vi "Main.vi"() -> ()   [LabVIEW 2013]
uses:
  Global.vi
  <userlib>/QLC/QLC.lvlib
panel:
  out "Error TCP_quad":errorcluster
  out "TCP_quad ID":refnum<k5>
  in  "Quadcopter":bool
  out "Trailers":bool[](array[boolean])
  out "Platooning Distance Scenario":dbl
  out "Distance2Master Scenario":dbl[](array[numeric])
  out "CurrentWP Final DarkGrey":i32
  out "Vref DarkGrey Final":dbl
  out "CurrentWP Final Grey":i32
  out "Vref Grey Final":dbl
  out "CurrentWP Final Black":i32
  out "Vref Black Final":dbl
  out "CurrentWP Final Blue":i32
  out "Vref Blue Final":dbl
  out "CurrentWP Final Red":i32
  out "Vref Red Final":dbl
  in  "Platooning Speed  Increment":dbl=1.25
  out "StopArrayOuter":i32[](array[numeric])
  out "StopArrayInner":i32[](array[numeric])
  out "PlatoonArray":i32[](array[numeric])
  out "Grey Truck Pose":sgl[](array[numeric])
  out "DarkGrey Truck Pose":dbl[](array[numeric])
  out "Current DarkGrey State":i32
  out "DarkGrey Trajectory WP Out":dbl[][](array[numeric])
  out "Red distance2Master DarkGrey":dbl
  out "DarkGrey dref":dbl
  out "Red distance2Master Grey":dbl
  out "Current Grey State":i32
  out "Grey Trajectory WP Out":dbl[][](array[numeric])
  out "Grey dref":dbl
  out "Change to state DarkGrey Scenario":i32
  out "Vref DarkGrey Scenario":dbl
  out "Change to state Grey Scenario":i32
  out "Vref Grey Scenario":dbl
  in  "ID DarkGrey":u8=5
  in  "ID Grey":u8=4
  in  "Change to state DarkGrey":i32(ring)=1 items=["Parking", "OuterLane", "InnerLane", "InnerRoad"]
  in  "Vref DarkGrey":dbl(slide) scale=0.0..1.5
  in  "Change to state Grey":i32(ring)=1 items=["Parking", "OuterLane", "InnerLane", "InnerRoad"]
  in  "Vref Grey":dbl(slide) scale=0.0..1.5
  out "X Grey":dbl
  out "Y  Grey":dbl
  out "Yaw  Grey":dbl
  out "X DarkGrey":dbl
  out "Y  DarkGrey":dbl
  out "Yaw  DarkGrey":dbl
  in  "ControllerGains DarkGrey":T1={"KPSteering"=1.0, "KDSteering"=0.0, "KPSpeed"=0.8, "KISpeed"=3.0, "KDSpeed"=0.2}
  out "Current state DarkGrey":i32(ring)=1 items=["Parking", "OuterLane", "InnerLane", "InnerRoad"]
  out "D2TL DarkGrey":dbl
  out "D2Master DarkGrey":dbl
  in  "With Trailer DarkGrey":bool
  out "Real Speed DarkGrey":dbl(knob) scale=0.0..2.0
  out "DarkGrey Speed":u8
  out "DarkGrey Steering":u8
  in  "ControllerGains Grey":T1={"KPSteering"=0.6, "KDSteering"=0.05, "KPSpeed"=0.8, "KISpeed"=3.0, "KDSpeed"=0.2}
  out "Current state Grey":i32(ring)=1 items=["Parking", "OuterLane", "InnerLane", "InnerRoad"]
  out "D2TL Grey":dbl
  out "D2Master Grey":dbl
  in  "With Trailer Grey":bool
  out "Real Speed Grey":dbl(knob) scale=0.0..2.0
  out "Grey Speed":u8
  out "Grey Steering":u8
  out "COM  DarkGrey":T2
  out "COM  Grey":T2
  in  "DarkGrey ID":u8=9
  in  "Grey ID":u8=8
  in  "Port DarkGrey":u16=9006
  in  "Port Grey":u16=9005
  in  "QTM ID DarkGrey":i32=3
  in  "QTM ID Grey":i32=5
  out "Vref":dbl[](array[numeric])
  out "bytes written 3":i32
  out "bytes written 2":i32
  out "ScenarioString":string
  out "red dref":dbl
  out "real distance2master red":dbl
  in  "ControllerGains Black":T1={"KPSteering"=0.9, "KDSteering"=0.05, "KPSpeed"=1.0, "KISpeed"=3.0, "KDSpeed"=0.2}
  in  "ControllerGains Blue":T1={"KPSteering"=1.0, "KDSteering"=0.05, "KPSpeed"=0.8, "KISpeed"=3.0, "KDSpeed"=0.2}
  out "Version":i32
  in  "Visualizer":bool
  out "Iter":i32
  out "NRoads":i32
  out "TL Outer Select":bool
  out "TL Inner Select":bool
  out "Error TCP":errorcluster
  out "TCP ID":refnum<k5>
  out "NTrucks":i32
  out "CurrentWP":i32[](array[numeric])
  out "Last QTM Event":dbl=2.0
  out "Change to state Red Scenario":i32
  out "Vref Red Scenario":dbl
  out "Change to state Blue Scenario":i32
  out "Vref Blue Scenario":dbl
  out "Change to state Black Scenario":i32
  out "Vref Black Scenario":dbl
  out "Ignore":bool
  out "Current state Red":i32(ring)=1 items=["Parking", "OuterLane", "InnerLane", "InnerRoad"]
  out "Current state Blue":i32(ring)=1 items=["Parking", "OuterLane", "InnerLane", "InnerRoad"]
  out "Current state Black":i32(ring)=1 items=["Parking", "OuterLane", "InnerLane", "InnerRoad"]
  in  "Tab Control":enum32{"Pedro Lima", "João Pedro Alvito"}(tab)
  in  "Scenario Selection PL":u32(ring) items=["Manual", "1 catch up 1", "1 catch up 2", "2 catch up 1", "1 catch up 1 from other road", "1 catch up 1 but master exits", "1 diferent mass catch up 2 without overtake", "1 different mass catch up 2 with overtake", "1 catch up 2 but middle leaves"]
  out "Info PL":string
  out "length":i32
  in  "Bridge":bool
  in  "Scenario Selection JPA":u32(ring) items=["Manual", "Simple traffic lights", "Simple anti-platoon", "Mixture", "Time Decision", "Timed Control with Platoon", "Anti-platoon"]
  out "Info JP":string
  out "X Red":dbl
  out "Y  Red":dbl
  out "Yaw  Red":dbl
  out "X Black":dbl
  out "Y Black":dbl
  out "Yaw Black":dbl
  out "Yaw Blue":dbl
  out "Y Blue":dbl
  out "X Blue":dbl
  out "D2TL Red":dbl
  out "D2TL Black":dbl
  out "D2TL Blue":dbl
  out "D2Master Red":dbl
  out "D2Master Black":dbl
  out "D2Master Blue":dbl
  out "Outer Red":bool
  out "Inner Green":bool
  out "Inner Red":bool
  out "Outer Green":bool
  out "D2TLFinal":dbl[](array[numeric])
  out "Truck Dimensions":dbl[](array[numeric])
  out "Traffic Lights":T3
  in  "Stop Button Inner":bool
  in  "Traffic Light Position Inner Lane":i32=23
  out "CurrentState":i32[](array[numeric])
  out "Real Speed Red":dbl(knob) scale=0.0..2.0
  out "Real Speed Black":dbl(knob) scale=0.0..2.0
  in  "Stop Button Outer":bool
  in  "Traffic Light Position Outer Lane":i32=27
  out "InnerRoad":T4
  out "Distance to Master":dbl[](array[numeric])
  out "Blue dref":dbl
  out "Blue distance2master blue":dbl
  out "black dref":dbl
  out "Red distance2Master black":dbl
  out "Red Trajectory WP Out":dbl[][](array[numeric])
  out "Blue Trajectory WP Out":dbl[][](array[numeric])
  out "Black Trajectory WP Out":dbl[][](array[numeric])
  in  "Change to state Black":i32(ring)=1 items=["Parking", "OuterLane", "InnerLane", "InnerRoad"]
  in  "Change to state Red":i32(ring)=1 items=["Parking", "OuterLane", "InnerLane", "InnerRoad"]
  out "Trajectory Network":T5(array[cluster])
  out "InnerLane":T4
  out "OuterLane":T4
  out "Current Red State":i32
  out "Current Black State":i32
  out "Current Blue State":i32
  in  "Change to state Blue":i32(ring)=1 items=["Parking", "OuterLane", "InnerLane", "InnerRoad"]
  out "Trucks Poses":dbl[][](array[numeric])
  out "Total Platooning Distance":dbl[](array[numeric])
  in  "With Trailer Red":bool
  in  "With Trailer  Black":bool
  in  "With Trailer Blue":bool
  in  "QTM ID Red":i32=4
  in  "QTM ID Blue":i32=2
  in  "QTM ID Black":i32=1
  in  "ID Black":u8=2
  in  "ID Red":u8=3
  in  "ID Blue":u8=1
  out "COM  Black":T2
  out "COM  Red":T2
  out "COM Blue":T2
  in  "Platooning Distance":dbl=0.3
  out "Distance2Master":dbl[](array[numeric])
  out "Real Speed Blue":dbl(knob) scale=0.0..2.0
  in  "Set MasterID":i32(ring) items=["None", "Blue Truck", "Black Truck", "Red Truck", "Grey Truck", "DarkGrey Truck"]
  in  "Vref Black":dbl(slide) scale=0.0..1.5
  in  "Vref Blue":dbl(slide) scale=0.0..1.5
  in  "Vref Red":dbl(slide) scale=0.0..1.5
  out "Red Truck Pose":dbl[](array[numeric])
  out "Blue Truck Pose":dbl[](array[numeric])
  out "Black Truck Pose":dbl[](array[numeric])
  out "Red Speed":u8
  out "Red Steering":u8
  in  "Event Label":string
  in  "Set Event":bool
  in  "stop":bool
  out "Blue Speed":u8
  out "Blue Steering":u8
  in  "Port Blue":u16=9002
  in  "Blue ID":u8=10
  out "Camera Timestamp":u64
  out "Camera Frame Number":u32
  in  "Control QTM":bool caption="Off   On"
  out "Controlling QTM":bool
  in  "Connect to QTM":bool=TRUE
  out "QTM Message":string
  in  "Data":string="6DEuler"
  in  "Frequency":string="AllFrames"
  in  "Port":i32=22222 min=22222 max=65535
  in  "Address":string="smlremote.no-ip.biz"
  in  "Port Red":u16=9004
  in  "Red ID":u8=7
  out "Black Speed":u8
  out "Black Steering":u8
  in  "Port Black":u16=9003
  in  "Black ID":u8=14
  in  "ControllerGains Red":T1={"KPSteering"=1.0, "KDSteering"=0.05, "KPSpeed"=0.8, "KISpeed"=3.0, "KDSpeed"=0.2}
types:
  T1 = cluster{"KPSteering":dbl, "KDSteering":dbl, "KPSpeed":dbl, "KISpeed":dbl, "KDSpeed":dbl}
  T2 = cluster{"Truck ID":u8, "connection ID":refnum<k5>}
  T3 = cluster{"Stop Button Outer":bool, "Stop WP Outer Lane":dbl, "Stop Button Inner":bool, "Stop WP Inner Lane ":dbl}
  T4 = cluster{"all rows":dbl[][], "all rows":dbl[][], "Array":i32[]}
  T5 = cluster{"Trajectory WP":dbl[][], "Distances LUT":dbl[][], "Trajectory length":i32[]}[]
  T6 = cluster{"pose":dbl[], "totalerror_v":dbl, "erroSteering":dbl, "ActualTime":dbl, "ActualTime 2":dbl}
  T7 = cluster{"all rows":dbl[][], "all rows":dbl[][], "Array":i32[]}[]
  T8 = cluster{"Trajectory WP":dbl[][], "Distances LUT":dbl[][], "Trajectory length":i32[]}
  T9 = cluster{"Vref Black":dbl, "Change to state Black":i32, "Vref Blue":dbl, "Change to state Blue":i32, "Vref Red":dbl, "Change to state Red":i32, "Vref Grey":dbl, "Change to state Grey":i32, "Vref DarkGrey":dbl, "Change to state DarkGrey":i32, "With Trailer Blue":bool, "With Trailer  Black":bool, "With Trailer Red":bool, "With Trailer Grey":bool, "With Trailer DarkGrey":bool, "Platooning Distance":dbl, "CurrentWP":i32[], "Distance to Master":dbl[], "D2TLFinal":dbl[], "CurrentState":i32[], "Trajectory Network":cluster{"Trajectory WP":dbl[][], "Distances LUT":dbl[][], "Trajectory length":i32[]}[]}
  T10 = cluster{"Vref_Black":dbl, "Change_to_state_Black":i32, "Vref_Blue":dbl, "Change_to_state_Blue":i32, "Vref_Red":dbl, "Change_to_state_Red":i32, "Vref_Grey":dbl, "Change_to_state_Grey":i32, "Vref_DarkGrey":dbl, "Change_to_state_DarkGrey":i32, "With_Trailer_Blue":bool, "With_Trailer_Black":bool, "With_Trailer_Red":bool, "With_Trailer_Grey":bool, "With_Trailer_DarkGrey":bool, "Platooning_Distance":dbl, "CurrentWP":i32[], "Distance2Master":dbl[], "d2TL":dbl[], "CurrentState":i32[], "TrajectoryNetwork":cluster{"TrajectoryWP":dbl[][], "DistancesLUT":dbl[][], "TrajectoryLength":i32[]}[]}
  T11 = cluster{"Stop Button Outer":bool, "Traffic Light Position Outer Lane":i32, "Stop Button Inner":bool, "Traffic Light Position Inner Lane":i32}
  T12 = cluster{"pose":dbl[], "totalerror_v":dbl, "erroSteering":dbl, "ActualTime":dbl, "error_v":dbl}
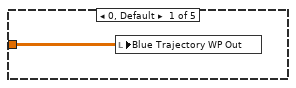
[diagram p5: hidden frame]
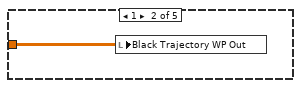
[diagram p6: hidden frame]
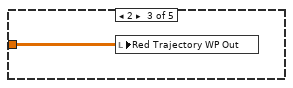
[diagram p7: hidden frame]
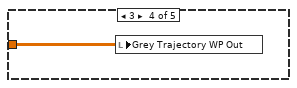
[diagram p8: hidden frame]
diagram:
  n1 = flat-sequence {
    frame #0 {
      n2 = flat-sequence {
        frame #0 {
          n3 = call "CreateConnection.vi"("Truck ID"="DarkGrey ID", "Port number\nactuators"="Port DarkGrey") -> ("COM data"=→"COM  DarkGrey":T2)  [unwired: 1 in]
          n4 = call "CreateConnection.vi"("Truck ID"="Red ID", "Port number\nactuators"="Port Red") -> ("COM data"=→"COM  Red":T2)  [unwired: 1 in]
          n5 = call "CreateConnection.vi"("Truck ID"="Black ID", "Port number\nactuators"="Port Black") -> ("COM data"=→"COM  Black":T2)  [unwired: 1 in]
          n6 = call "CreateConnection.vi"("Truck ID"="Blue ID", "Port number\nactuators"="Port Blue") -> ("COM data"=→"COM Blue":T2)  [unwired: 1 in]
          n7 = call "CreateConnection.vi"("Truck ID"="Grey ID", "Port number\nactuators"="Port Grey") -> ("COM data"=→"COM  Grey":T2)  [unwired: 1 in]
        }
      }
      n8 = flat-sequence {
        frame #0 {
          # "Initializations"
          n9 = Build Array(0 ("element"), 0 ("element"), 0 ("element"), 0 ("element"), 0 ("element")) -> (w78:i32[])
          "CurrentState" <- w78
          n10 = Build Array(0 ("element"), 0 ("element"), 0 ("element"), 0 ("element"), 0 ("element")) -> (→"CurrentWP":i32[])
          n11 = global write "Global.vi" "Transition WP"(i32[][] [[-1, -1, -1, -1], [-1, -1, -1, -1], [-1, -1, 5, 1], [-1, -1, 50, 25]] ("Transition WP")) -> ()
          n12 = global write "Global.vi" "RealSpeed"(dbl[] [] ("RealSpeed")) -> ()
          n13 = Build Array("Tab Control", "Scenario Selection PL", "Scenario Selection JPA") -> (w59:u32[])
          n14 = global write "Global.vi" "ScenarioArray"(w59) -> ()
          n15 = Array Size(array=w78) -> (size(s)=→"NTrucks":i32)
          n16 = local write "Set MasterID"(0 ("MasterID")) -> ()
          n17 = global write "Global.vi" "IsOvertaking"(FALSE ("IsOvertaking")) -> ()
          n18 = Index Array(array=w59, index=0) -> (element=w60:u32)
          n19 = global write "Global.vi" "Positioned"(FALSE ("FirstTime")) -> ()
          n20 = global write "Global.vi" "MasterID"(0 ("MasterID")) -> ()
          n21 = Increment(x=w60) -> (x+1=w61:u32)
          n22 = global write "Global.vi" "stop"(FALSE ("stop")) -> ()
          n23 = Index Array(array=w59, index=w61) -> (element=w62:u32)
          n24 = global write "Global.vi" "TL  Inner"(FALSE ("TL  Inner")) -> ()
          n25 = global write "Global.vi" "TL Outer"(FALSE ("TL Outer")) -> ()
          n26 = global write "Global.vi" "Lap Counter"(0 ("Lap Counter")) -> ()
          n27 = global write "Global.vi" "FirstTime"(TRUE ("FirstTime")) -> ()
          n28 = Not Equal To 0?(x=w62) -> (x != 0?=→"Ignore":bool)
          n29 = global write "Global.vi" "SetMasterID"(0 ("MasterID")) -> ()
          "ScenarioString" <- " " ("ScenarioString")
          "Vref" <- dbl[] [] ("RealSpeed")
        }
      }
      n30 = flat-sequence {
        frame #0 {
          n31 = local read "Tab Control"() -> (w2:enum32{"Pedro Lima", "João Pedro Alvito"})
          n32 = call "GetVersion.vi"() -> ("number"=→"Version":i32)
          n33 = Not Equal To 0?(x=w2) -> (x != 0?=w1:bool)
          n34 = local read "Version"() -> (w7:i32)
          n35 = local read "Version"() -> (w8:i32)
          n36 = local read "Version"() -> (w9:i32)
          n37 = local read "Version"() -> (w10:i32)
          n38 = local read "Version"() -> (w12:i32)
          n39 = local read "Version"() -> (w14:i32)
          n40 = local read "Version"() -> (w6:i32)
          n41 = local read "Version"() -> (w13:i32)
          n42 = call "CreatePath.vi"("Matlab Version"=w7, "filename"="OuterLaneBridgeLUT.txt") -> ("FinalPath"=w20:path)
          n43 = call "CreatePath.vi"("Matlab Version"=w8, "filename"="OuterLaneLUT.txt") -> ("FinalPath"=w22:path)
          n44 = call "CreatePath.vi"("Matlab Version"=w9, "filename"="OuterLaneBridge.txt") -> ("FinalPath"=w24:path)
          n45 = call "CreatePath.vi"("Matlab Version"=w10, "filename"="OuterLane.txt") -> ("FinalPath"=w26:path)
          n46 = call "CreatePath.vi"("Matlab Version"=w12, "filename"="InnerLaneBridgeLUT.txt") -> ("FinalPath"=w34:path)
          n47 = call "CreatePath.vi"("Matlab Version"=w14, "filename"="InnerLaneLUT.txt") -> ("FinalPath"=w33:path)
          n48 = call "CreatePath.vi"("Matlab Version"=w6, "filename"="InnerLaneBridge.txt") -> ("FinalPath"=w30:path)
          n49 = call "CreatePath.vi"("Matlab Version"=w13, "filename"="InnerLane.txt") -> ("FinalPath"=w28:path)
          n50 = local read "Version"() -> (w11:i32)
          n51 = local read "Version"() -> (w15:i32)
          n52 = And(x="Bridge", y=w1) -> (x .and. y?=w4:bool)
          n53 = call "CreatePath.vi"("Matlab Version"=w11, "filename"="InnerRoadLUT.txt") -> ("FinalPath"=w16:path)
          n54 = call "CreatePath.vi"("Matlab Version"=w15, "filename"="InnerRoad.txt") -> ("FinalPath"=w18:path)
          n55 = Select(t=w20, s=w4, f=w22) -> (s? t:f=w41:path)
          n56 = Select(t=w24, s=w4, f=w26) -> (s? t:f=w40:path)
          n57 = Select(t=w34, s=w4, f=w33) -> (s? t:f=w38:path)
          n58 = Select(t=w30, s=w4, f=w28) -> (s? t:f=w39:path)
          n59 = call "ReadFromFile.vi"("Trajectory Path File"=w40, "Trajectory Distances LUT"=w41) -> ("Trajectory Data"=w45:T4)  [unwired: 1 in]
          "OuterLane" <- w45
          n60 = call "ReadFromFile.vi"("Trajectory Path File"=w18, "Trajectory Distances LUT"=w16) -> ("Trajectory Data"=w42:T4)  [unwired: 1 in]
          "InnerRoad" <- w42
          n61 = call "ReadFromFile.vi"("Trajectory Path File"=w39, "Trajectory Distances LUT"=w38) -> ("Trajectory Data"=w44:T4)  [unwired: 1 in]
          "InnerLane" <- w44
          n62 = Build Array(T4 {"all rows"=[], "all rows"=[], "Array"=[]} ("element"), w45, w44, w42) -> (w37:T7)
          "Trajectory Network" <- w37
          n63 = Array Size(array=w37) -> (size(s)=→"NRoads":i32)
        }
      }
    }
    frame #1 {
      n64 = local read "Visualizer"() -> (w98:bool)
      n65 = local read "Quadcopter"() -> (w97:bool)
      n66 = case shown="True" w98 {
        frame False {
        }
        frame True {
          n67 = flat-sequence {
            frame #0 {
              n68 = local read "Trajectory Network"() -> (w109:T5)
              n69 = Index Array(array=w109) -> (element #2=w110:T8, element #3=w111:T8, element #4=w112:T8)  [unwired: 4 in, 1 out]
              n70 = Unbundle By Name(w110) -> ("Trajectory length"=w116:i32[], "Trajectory WP"=w124:dbl[][])
              n71 = Unbundle By Name(w111) -> ("Trajectory length"=w120:i32[], "Trajectory WP"=w125:dbl[][])
              n72 = Unbundle By Name(w112) -> ("Trajectory length"=w121:i32[], "Trajectory WP"=w126:dbl[][])
              n73 = Index Array(array=w116, index=0) -> (element=w127:i32)
              n74 = Index Array(array=w120, index=0) -> (element=w129:i32)
              n75 = Index Array(array=w121, index=0) -> (element=w131:i32)
              n76 = local read "NRoads"() -> (w138:i32)
              n77 = Multiply(x=w127, y=2) -> (x*y=w122:i32)
              n78 = Multiply(x=w129, y=2) -> (x*y=w123:i32)
              n79 = Multiply(x=w131, y=2) -> (x*y=w103:i32)
              n80 = Reshape Array(w124, w122) -> (w128:dbl[])
              n81 = Reshape Array(w125, w123) -> (w130:dbl[])
              n82 = Reshape Array(w126, w103) -> (w132:dbl[])
              n83 = Subtract(x=w138, y=1) -> (x-y=w139:i32)
              n84 = Build Array (concatenate)(w139, w127, w128, w129, w130, w131, w132) -> (w106:dbl[])
              n85 = To Double Precision Float(number=w106) -> (double precision float=w107:dbl[])
              n86 = Type Cast(x=w107) -> (*(type *) &x=w108:string)  [unwired: 1 in]
              n87 = call <vilib>:"TCP Listen.vi"("timeout ms (wait forever: -1)"=-1, "port"=u16 55000 ("remote port or service name")) -> ("error out"=w134:errorcluster, "connection ID"=w133:refnum<k5>)  [unwired: 5 in, 3 out]
              n88 = TCP Write(connection ID=w133, data in=w108, error in (no error)=w134) -> (connection ID out=→"TCP ID":refnum<k5>, error out=→"Error TCP":errorcluster)  [unwired: 1 in, 1 out]
            }
            frame #1 {
              n89 = local read "Bridge"() -> (w141:bool)
              n90 = Boolean To (0,1)(Boolean=w141) -> (0, 1=w140:i16)
              n91 = global read "Global.vi" "ScenarioArray"() -> (w143:u32[])
              n92 = local read "NTrucks"() -> (w142:i32)
              n93 = Build Array (concatenate)(w143, w142, w140) -> (w145:u32[])
              n94 = To Double Precision Float(number=w145) -> (double precision float=w144:dbl[])
              n95 = Type Cast(x=w144) -> (*(type *) &x=w146:string)  [unwired: 1 in]
              n96 = local read "Error TCP"() -> (w148:errorcluster)
              n97 = local read "TCP ID"() -> (w147:refnum<k5>)
              n98 = TCP Write(connection ID=w147, data in=w146, error in (no error)=w148) -> (connection ID out=w150:refnum<k5>, error out=w149:errorcluster)  [unwired: 1 in, 1 out]
              n99 = local write "TCP ID"(w150) -> ()
              n100 = local write "Error TCP"(w149) -> ()
            }
          }
        }
      }
      n101 = case shown="True" w97 {
        frame False {
        }
        frame True {
          n102 = call <vilib>:"TCP Listen.vi"("timeout ms (wait forever: -1)"=-1, "port"=u16 56999 ("remote port or service name")) -> ("error out"=→"Error TCP_quad":errorcluster, "connection ID"=→"TCP_quad ID":refnum<k5>)  [unwired: 5 in, 3 out]
        }
      }
    }
    frame #2 {
      n103 = while {
        stop <- w574 stop-if-true
        n104 = global read "Global.vi" "stop"() -> (w571:bool)
        n105 = call <userlib>:"Q Command.vi"("pEventLabel"="Event Label", "bEvent"="Set Event") -> ()  [unwired: 13 in, 1 out]
        n106 = Select(t=FALSE, s=w571, f="Connect to QTM") -> (s? t:f=w568:bool)
        n107 = call <userlib>:"QLC.vi"("connect"=w568, "data"="Data", "address"="Address", "port"="Port", "frequency"="Frequency", "controlQTM"="Control QTM") -> ("camFrameNumber"=→"Camera Frame Number":u32, "message"=→"QTM Message":string, "lastEvent"=→"Last QTM Event":i32, "QTMMaster"=→"Controlling QTM":bool, "camTimeStamp"=→"Camera Timestamp":u64)  [unwired: 4 in, 1 out]
        n108 = global read "Global.vi" "stop"() -> (w574:bool)
      }
      n109 = while {
        i -> [w151]
        stop <- "stop" stop-if-true
        n110 = flat-sequence {
          frame #0 {
            n111 = call "GetPose.vi"("QTM ID"="QTM ID Blue") -> ("Pose"=w162:sgl[])  [unwired: 10 in]
            "Blue Truck Pose" <- w162
            n112 = call "GetPose.vi"("QTM ID"="QTM ID Grey") -> ("Pose"=w158:sgl[])  [unwired: 10 in]
            "Grey Truck Pose" <- w158
            n113 = call "GetPose.vi"("QTM ID"="QTM ID DarkGrey") -> ("Pose"=w156:sgl[])  [unwired: 10 in]
            "DarkGrey Truck Pose" <- w156
            n114 = call "GetPose.vi"("QTM ID"="QTM ID Black") -> ("Pose"=w160:sgl[])  [unwired: 10 in]
            "Black Truck Pose" <- w160
            n115 = call "GetPose.vi"("QTM ID"="QTM ID Red") -> ("Pose"=w154:sgl[])  [unwired: 10 in]
            "Red Truck Pose" <- w154
            n116 = Build Array(w162, w160, w154, w158, w156) -> (→"Trucks Poses":sgl[][])
            n117 = Index Array(array=w162) -> (element #1=→"X Blue":sgl, element #2=→"Y Blue":sgl, element #3=→"Yaw Blue":sgl)  [unwired: 3 in]
            n118 = Index Array(array=w160) -> (element #1=→"X Black":sgl, element #2=→"Y Black":sgl, element #3=→"Yaw Black":sgl)  [unwired: 3 in]
            n119 = Index Array(array=w158) -> (element #1=→"X Grey":sgl, element #2=→"Y  Grey":sgl, element #3=→"Yaw  Grey":sgl)  [unwired: 3 in]
            n120 = Index Array(array=w156) -> (element #1=→"X DarkGrey":sgl, element #2=→"Y  DarkGrey":sgl, element #3=→"Yaw  DarkGrey":sgl)  [unwired: 3 in]
            n121 = Index Array(array=w154) -> (element #1=→"X Red":sgl, element #2=→"Y  Red":sgl, element #3=→"Yaw  Red":sgl)  [unwired: 3 in]
          }
          frame #1 {
            w191 = 0.5 ("t")
            w192 = 1.3 ("t")
            n122 = local read "Trajectory Network"() -> (w205:T5)
            n123 = local read "Distance to Master"() -> (w208:dbl[])
            n124 = local read "CurrentState"() -> (w206:i32[])
            n125 = local read "CurrentWP"() -> (w209:i32[])
            n126 = local read "D2TLFinal"() -> (w207:dbl[])
            n127 = Bundle("Vref Black"="Vref Black", "Change to state Black"="Change to state Black", "Vref Blue"="Vref Blue", "Change to state Blue"="Change to state Blue", "Vref Red"="Vref Red", "Change to state Red"="Change to state Red", "Vref Grey"="Vref Grey", "Change to state Grey"="Change to state Grey", "Vref DarkGrey"="Vref DarkGrey", "Change to state DarkGrey"="Change to state DarkGrey", "With Trailer Blue"="With Trailer Blue", "With Trailer  Black"="With Trailer  Black", "With Trailer Red"="With Trailer Red", "With Trailer Grey"="With Trailer Grey", "With Trailer DarkGrey"="With Trailer DarkGrey", "Platooning Distance"="Platooning Distance", "CurrentWP"=w209, "Distance to Master"=w208, "D2TLFinal"=w207, "CurrentState"=w206, "Trajectory Network"=w205) -> (w197:T9)  [unwired: 1 in]
            n128 = call "ScenarioScript.vi"("Control In"=w197) -> ("Control Out"=w217:T10, "String"=w204:string)
            "Info PL" <- w204
            "Info JP" <- w204
            n129 = local write "ScenarioString"(w204) -> ()
            n130 = Unbundle By Name(w217) -> ("Vref_Black"=→"Vref Black Scenario":dbl, "Change_to_state_Black"=→"Change to state Black Scenario":i32, "Vref_Blue"=→"Vref Blue Scenario":dbl, "Change_to_state_Blue"=→"Change to state Blue Scenario":i32, "Vref_Red"=→"Vref Red Scenario":dbl, "Change_to_state_Red"=→"Change to state Red Scenario":i32, "Vref_Grey"=→"Vref Grey Scenario":dbl, "Change_to_state_Grey"=→"Change to state Grey Scenario":i32, "Vref_DarkGrey"=→"Vref DarkGrey Scenario":dbl, "Change_to_state_DarkGrey"=→"Change to state DarkGrey Scenario":i32, "With_Trailer_Blue"=w185:bool, "With_Trailer_Black"=w184:bool, "With_Trailer_Red"=w183:bool, "With_Trailer_Grey"=w182:bool, "With_Trailer_DarkGrey"=w181:bool, "Platooning_Distance"=w211:dbl, "Distance2Master"=w188:dbl[])
            "Platooning Distance Scenario" <- w211
            n131 = Select(t=w192, s=w185, f=w191) -> (s? t:f=w228:dbl)
            n132 = Select(t=w192, s=w184, f=w191) -> (s? t:f=w229:dbl)
            n133 = Select(t=w192, s=w183, f=w191) -> (s? t:f=w230:dbl)
            n134 = Select(t=w192, s=w182, f=w191) -> (s? t:f=w190:dbl)
            n135 = Select(t=w192, s=w181, f=w191) -> (s? t:f=w189:dbl)
            n136 = Build Array(w185, w184, w183, w182, w181) -> (→"Trailers":bool[])
            n137 = Build Array(w228, w229, w230, w190, w189) -> (w187:dbl[])
            "Truck Dimensions" <- w187
            n138 = Add(x=w187, y=w211) -> (x+y=→"Total Platooning Distance":dbl[])
            n139 = Add(x=w188, y=w187) -> (x+y=→"Distance2Master Scenario":dbl[])
          }
          frame #2 {
            n140 = local read "Change to state DarkGrey Scenario"() -> (w279:i32)
            n141 = local read "Change to state Black Scenario"() -> (w302:i32)
            n142 = local read "Change to state Grey Scenario"() -> (w292:i32)
            n143 = local read "Change to state Blue Scenario"() -> (w301:i32)
            n144 = local read "Platooning Speed  Increment"() -> (w262:dbl)
            n145 = local read "Platooning Speed  Increment"() -> (w266:dbl)
            n146 = local read "Platooning Speed  Increment"() -> (w265:dbl)
            n147 = local read "Change to state Red Scenario"() -> (w303:i32)
            n148 = local read "Platooning Speed  Increment"() -> (w264:dbl)
            n149 = local read "Platooning Speed  Increment"() -> (w263:dbl)
            n150 = local read "Total Platooning Distance"() -> (w312:dbl[])
            n151 = local read "Distance2Master Scenario"() -> (w326:dbl[])
            n152 = local read "Total Platooning Distance"() -> (w288:dbl[])
            n153 = local read "Distance2Master Scenario"() -> (w284:dbl[])
            n154 = local read "Total Platooning Distance"() -> (w275:dbl[])
            n155 = local read "Distance2Master Scenario"() -> (w271:dbl[])
            n156 = local read "Total Platooning Distance"() -> (w328:dbl[])
            n157 = local read "Distance2Master Scenario"() -> (w327:dbl[])
            n158 = local read "Total Platooning Distance"() -> (w316:dbl[])
            n159 = local read "Distance2Master Scenario"() -> (w317:dbl[])
            n160 = local read "Vref DarkGrey Scenario"() -> (w252:dbl)
            n161 = local read "Real Speed DarkGrey"() -> (w267:dbl)
            n162 = local read "Trajectory Network"() -> (w314:T5)
            n163 = local read "Trajectory Network"() -> (w286:T5)
            n164 = local read "Trajectory Network"() -> (w273:T5)
            n165 = local read "Trajectory Network"() -> (w333:T5)
            n166 = local read "Trajectory Network"() -> (w319:T5)
            n167 = local read "Vref Black Scenario"() -> (w254:dbl)
            n168 = local read "Vref Grey Scenario"() -> (w253:dbl)
            n169 = local read "Vref Red Scenario"() -> (w256:dbl)
            n170 = local read "Vref Blue Scenario"() -> (w255:dbl)
            n171 = local read "Real Speed Black"() -> (w325:dbl)
            n172 = local read "Real Speed Blue"() -> (w337:dbl)
            n173 = local read "Real Speed Grey"() -> (w268:dbl)
            n174 = local read "Real Speed Red"() -> (w324:dbl)
            n175 = local read "PlatoonArray"() -> (w234:i32[])
            n176 = local read "Traffic Lights"() -> (w320:T3)
            n177 = local read "PlatoonArray"() -> (w233:i32[])
            n178 = local read "Traffic Lights"() -> (w285:T3)
            n179 = local read "PlatoonArray"() -> (w232:i32[])
            n180 = local read "Traffic Lights"() -> (w272:T3)
            n181 = local read "PlatoonArray"() -> (w236:i32[])
            n182 = local read "Traffic Lights"() -> (w321:T3)
            n183 = local read "PlatoonArray"() -> (w235:i32[])
            n184 = local read "Traffic Lights"() -> (w322:T3)
            n185 = local read "Trucks Poses"() -> (w313:dbl[][])
            n186 = local read "Trucks Poses"() -> (w287:dbl[][])
            n187 = local read "Trucks Poses"() -> (w274:dbl[][])
            n188 = local read "Trucks Poses"() -> (w331:dbl[][])
            n189 = local read "Trucks Poses"() -> (w329:dbl[][])
            n190 = local read "CurrentState"() -> (w310:i32[])
            n191 = local read "Set MasterID"() -> (w259:i32)
            n192 = local read "CurrentState"() -> (w290:i32[])
            n193 = local read "Set MasterID"() -> (w260:i32)
            n194 = local read "CurrentState"() -> (w277:i32[])
            n195 = local read "Set MasterID"() -> (w261:i32)
            n196 = local read "CurrentState"() -> (w323:i32[])
            n197 = local read "Set MasterID"() -> (w257:i32)
            n198 = local read "CurrentState"() -> (w315:i32[])
            n199 = local read "Set MasterID"() -> (w258:i32)
            n200 = local read "ID DarkGrey"() -> (w276:u8)
            n201 = local read "CurrentWP"() -> (w249:i32[])
            n202 = local read "CurrentWP"() -> (w248:i32[])
            n203 = local read "CurrentWP"() -> (w247:i32[])
            n204 = local read "CurrentWP"() -> (w251:i32[])
            n205 = local read "CurrentWP"() -> (w250:i32[])
            n206 = local read "D2TLFinal"() -> (w307:dbl[])
            n207 = local read "D2TLFinal"() -> (w291:dbl[])
            n208 = local read "D2TLFinal"() -> (w278:dbl[])
            n209 = local read "D2TLFinal"() -> (w309:dbl[])
            n210 = local read "D2TLFinal"() -> (w308:dbl[])
            n211 = local read "ID Black"() -> (w311:u8)
            n212 = local read "ID Grey"() -> (w289:u8)
            n213 = local read "ID Blue"() -> (w318:u8)
            n214 = local read "ID Red"() -> (w332:u8)
            n215 = call "DecisionMaker.vi"("Trajectory Network"=w314, "Change to state"=w302, "Vref"=w254, "K"=w262, "Platooning distances"=w312, "Current State In"=w310, "Set MasterID"=w259, "Current WP In"=w249, "MyID"=w311, "Distance2Master"=w326, "PlatoonArray"=w234, "Traffic Lights"=w320, "Trucks Poses"=w313, "d2TLFinal"=w307) -> ("d"=→"Red distance2Master black":dbl, "dref"=→"black dref":dbl, "Current State Out"=→"Current Black State" →"Current state Black":i32, "VrefOut"=→"Vref Black Final":dbl, "CurrentWPOut"=→"CurrentWP Final Black":i32, "Trajectory WP Out"=→"Black Trajectory WP Out":dbl[][])  [unwired: 8 in]
            n216 = call "DecisionMaker.vi"("Trajectory Network"=w286, "Change to state"=w292, "Vref"=w253, "K"=w266, "Platooning distances"=w288, "Current State In"=w290, "Set MasterID"=w260, "Current WP In"=w248, "MyID"=w289, "Distance2Master"=w284, "PlatoonArray"=w233, "Traffic Lights"=w285, "Trucks Poses"=w287, "d2TLFinal"=w291) -> ("d"=→"Red distance2Master Grey":dbl, "dref"=→"Grey dref":dbl, "Current State Out"=→"Current Grey State" →"Current state Grey":i32, "VrefOut"=→"Vref Grey Final":dbl, "CurrentWPOut"=→"CurrentWP Final Grey":i32, "Trajectory WP Out"=→"Grey Trajectory WP Out":dbl[][])  [unwired: 8 in]
            n217 = call "DecisionMaker.vi"("Trajectory Network"=w273, "Change to state"=w279, "Vref"=w252, "K"=w265, "Platooning distances"=w275, "Current State In"=w277, "Set MasterID"=w261, "Current WP In"=w247, "MyID"=w276, "Distance2Master"=w271, "PlatoonArray"=w232, "Traffic Lights"=w272, "Trucks Poses"=w274, "d2TLFinal"=w278) -> ("d"=→"Red distance2Master DarkGrey":dbl, "dref"=→"DarkGrey dref":dbl, "Current State Out"=→"Current state DarkGrey" →"Current DarkGrey State":i32, "VrefOut"=→"Vref DarkGrey Final":dbl, "CurrentWPOut"=→"CurrentWP Final DarkGrey":i32, "Trajectory WP Out"=→"DarkGrey Trajectory WP Out":dbl[][])  [unwired: 8 in]
            n218 = call "DecisionMaker.vi"("Trajectory Network"=w333, "Change to state"=w303, "Vref"=w256, "K"=w264, "Platooning distances"=w328, "Current State In"=w323, "Set MasterID"=w257, "Current WP In"=w251, "MyID"=w332, "Distance2Master"=w327, "PlatoonArray"=w236, "Traffic Lights"=w321, "Trucks Poses"=w331, "d2TLFinal"=w309) -> ("d"=→"real distance2master red":dbl, "dref"=→"red dref":dbl, "Current State Out"=→"Current Red State" →"Current state Red":i32, "VrefOut"=→"Vref Red Final":dbl, "CurrentWPOut"=→"CurrentWP Final Red":i32, "Trajectory WP Out"=→"Red Trajectory WP Out":dbl[][])  [unwired: 8 in]
            n219 = call "DecisionMaker.vi"("Trajectory Network"=w319, "Change to state"=w301, "Vref"=w255, "K"=w263, "Platooning distances"=w316, "Current State In"=w315, "Set MasterID"=w258, "Current WP In"=w250, "MyID"=w318, "Distance2Master"=w317, "PlatoonArray"=w235, "Traffic Lights"=w322, "Trucks Poses"=w329, "d2TLFinal"=w308) -> ("d"=→"Blue distance2master blue":dbl, "dref"=→"Blue dref":dbl, "Current State Out"=→"Current Blue State" →"Current state Blue":i32, "VrefOut"=→"Vref Blue Final":dbl, "CurrentWPOut"=→"CurrentWP Final Blue":i32, "Trajectory WP Out"=→"Blue Trajectory WP Out":dbl[][])  [unwired: 8 in]
            n220 = Build Array(w337, w325, w324, w268, w267) -> (w330:dbl[])
            n221 = global write "Global.vi" "RealSpeed"(w330) -> ()
          }
          frame #3 {
            n222 = flat-sequence {
              frame #0 {
                n223 = local read "CurrentWP Final DarkGrey"() -> (w366:i32)
                n224 = local read "Current DarkGrey State"() -> (w351:i32)
                n225 = local read "CurrentWP Final Black"() -> (w364:i32)
                n226 = local read "CurrentWP Final Blue"() -> (w363:i32)
                n227 = local read "CurrentWP Final Grey"() -> (w367:i32)
                n228 = local read "CurrentWP Final Red"() -> (w365:i32)
                n229 = local read "Current Black State"() -> (w353:i32)
                n230 = local read "Vref DarkGrey Final"() -> (w357:dbl)
                n231 = local read "Current Grey State"() -> (w350:i32)
                n232 = local read "Current Blue State"() -> (w354:i32)
                n233 = local read "Current Red State"() -> (w352:i32)
                n234 = local read "Vref Black Final"() -> (w359:dbl)
                n235 = local read "Vref Grey Final"() -> (w356:dbl)
                n236 = local read "Vref Blue Final"() -> (w360:dbl)
                n237 = local read "Vref Red Final"() -> (w358:dbl)
                n238 = Build Array(w354, w353, w352, w350, w351) -> (w355:i32[])
                n239 = Build Array(w363, w364, w365, w367, w366) -> (w362:i32[])
                n240 = Build Array(w360, w359, w358, w356, w357) -> (w361:dbl[])
                n241 = local write "CurrentState"(w355) -> ()
                n242 = local write "CurrentWP"(w362) -> ()
                n243 = local write "Vref"(w361) -> ()
              }
              frame #1 {
                n244 = global read "Global.vi" "SetMasterID"() -> (w371:i32)
                n245 = local read "Ignore"() -> (w372:bool)
                n246 = Select(t=w371, s=w372, f="Set MasterID") -> (s? t:f=w368:i32)
                n247 = local write "Set MasterID"(w368) -> ()
                n248 = case shown="1, Default" w368 {
                  selector: w368 -> [w373 w378]
                  tunnel: [w373 w377] -> w369
                  frame 0 {
                  }
                  frame 1, Default {
                    n249 = local read "Total Platooning Distance"() -> (w374:dbl[])
                    n250 = local read "Trajectory Network"() -> (w380:T5)
                    n251 = local read "PlatoonArray"() -> (w382:i32[])
                    n252 = local read "Trucks Poses"() -> (w381:dbl[][])
                    n253 = local read "CurrentState"() -> (w379:i32[])
                    n254 = local read "CurrentWP"() -> (w376:i32[])
                    n255 = local read "Vref"() -> (w383:dbl[])
                    n256 = call "OvertakingDecisor.vi"("Trajectory Network"=w380, "PlatoonArray"=w382, "Trucks Poses"=w381, "Current State In"=w379, "Total Platooning Distance"=w374, "Set MasterID"=w378, "CurrentWP"=w376, "Vref"=w383) -> ("VrefOut"=w389:dbl, "Current WP Out"=w388:i32, "Set MasterID Out"=w377:i32, "Current State Out"=w387:i32, "Trajectory WP Out"=w393:dbl[][])  [unwired: 3 in]
                    n257 = Decrement(x=w378) -> (x-1=w392:i32)
                    n258 = local read "CurrentState"() -> (w386:i32[])
                    n259 = case shown="4" w392 {
                      tunnel: w393 -> [w394 w395 w396 w397 w398]
                      frame 0, Default {
                        n260 = local write "Blue Trajectory WP Out"(w394) -> ()
                      }
                      frame 1 {
                        n261 = local write "Black Trajectory WP Out"(w395) -> ()
                      }
                      frame 2 {
                        n262 = local write "Red Trajectory WP Out"(w396) -> ()
                      }
                      frame 3 {
                        n263 = local write "Grey Trajectory WP Out"(w397) -> ()
                      }
                      frame 4 {
                        n264 = local write "DarkGrey Trajectory WP Out"(w398) -> ()
                      }
                    }
                    n265 = local read "CurrentWP"() -> (w384:i32[])
                    n266 = local read "Vref"() -> (w385:dbl[])
                    n267 = Replace Array Subset(array=w385, new element=w389, index=w392) -> (w390:dbl[])
                    n268 = Replace Array Subset(array=w384, new element=w388, index=w392) -> (w391:i32[])
                    n269 = Replace Array Subset(array=w386, new element=w387, index=w392) -> (w375:i32[])
                    n270 = local write "Vref"(w390) -> ()
                    n271 = local write "CurrentWP"(w391) -> ()
                    n272 = local write "CurrentState"(w375) -> ()
                  }
                }
                n273 = global write "Global.vi" "MasterID"(w369) -> ()
              }
            }
            n274 = global read "Global.vi" "TL Outer"() -> (w344:bool)
            n275 = global read "Global.vi" "TL  Inner"() -> (w342:bool)
            n276 = local read "Ignore"() -> (w340:bool)
            n277 = Select(t=w344, s=w340, f="Stop Button Outer") -> (s? t:f=w338:bool)
            "Outer Red" <- w338
            "TL Outer Select" <- w338
            n278 = Select(t=w342, s=w340, f="Stop Button Inner") -> (s? t:f=w339:bool)
            "Inner Red" <- w339
            "TL Inner Select" <- w339
            n279 = Bundle("Stop Button Outer"=w338, "Traffic Light Position Outer Lane"="Traffic Light Position Outer Lane", "Stop Button Inner"=w339, "Traffic Light Position Inner Lane"="Traffic Light Position Inner Lane") -> (→"Traffic Lights":T11)  [unwired: 1 in]
            n280 = Not(x=w338) -> (.not. x?=→"Outer Green":bool)
            n281 = Not(x=w339) -> (.not. x?=→"Inner Green":bool)
          }
          frame #4 {
            n282 = local read "Trajectory Network"() -> (w418:T5)
            n283 = local read "Truck Dimensions"() -> (w416:dbl[])
            n284 = local read "Traffic Lights"() -> (w417:T3)
            n285 = local read "Trucks Poses"() -> (w419:dbl[][])
            n286 = local read "CurrentState"() -> (w420:i32[])
            n287 = local read "CurrentWP"() -> (w407:i32[])
            n288 = global read "Global.vi" "MasterID"() -> (w424:i32)
            n289 = local read "Trajectory Network"() -> (w428:T5)
            n290 = call "GetDistance2TL.vi"("Traffic Lights"=w417, "Truck Dimensions"=w416, "Trajectory Network"=w418, "CurrentWP"=w407, "Trucks Poses"=w419, "Current State"=w420) -> ("StopArray_2"=→"StopArrayInner":i32[], "d2TLFinal"=w411:dbl[], "StopArray_1"=→"StopArrayOuter":i32[])
            "D2TLFinal" <- w411
            n291 = local read "Trucks Poses"() -> (w421:dbl[][])
            n292 = local read "Set MasterID"() -> (w399:i32)
            n293 = Subtract(x=w424, y=1) -> (x-y=w427:i32)
            n294 = local read "Truck Dimensions"() -> (w423:dbl[])
            n295 = local read "CurrentState"() -> (w429:i32[])
            n296 = call "GetDistance2Master.vi"("TrucksPoses"=w421, "Set MasterID"=w399, "Trajectory Network"=w428, "Current State"=w429) -> ("Distance2Master"=w422:dbl[], "PlatoonArray"=→"PlatoonArray":i32[])
            "Distance2Master" <- w422
            n297 = Index Array(array=w423, index=w427) -> (element=w425:dbl)
            n298 = Index Array(array=w411) -> (element #1=→"D2TL Blue":dbl, element #2=→"D2TL Black":dbl, element #3=→"D2TL Red":dbl, element #4=→"D2TL Grey":dbl, element #5=→"D2TL DarkGrey":dbl)  [unwired: 5 in]
            n299 = Subtract(x=w422, y=w425) -> (x-y=w415:dbl[])
            "Distance to Master" <- w415
            n300 = Index Array(array=w415) -> (element #1=→"D2Master Blue":dbl, element #2=→"D2Master Black":dbl, element #3=→"D2Master Red":dbl, element #4=→"D2Master Grey":dbl, element #5=→"D2Master DarkGrey":dbl)  [unwired: 5 in]
          }
          frame #5 {
            n301 = local read "DarkGrey Trajectory WP Out"() -> (w454:dbl[][])
            n302 = local read "Black Trajectory WP Out"() -> (w478:dbl[][])
            n303 = local read "Blue Trajectory WP Out"() -> (w487:dbl[][])
            n304 = local read "Grey Trajectory WP Out"() -> (w467:dbl[][])
            n305 = local read "Red Trajectory WP Out"() -> (w493:dbl[][])
            n306 = local read "DarkGrey Truck Pose"() -> (w458:dbl[])
            n307 = local read "Black Truck Pose"() -> (w503:dbl[])
            n308 = local read "Grey Truck Pose"() -> (w459:sgl[])
            n309 = local read "Blue Truck Pose"() -> (w489:dbl[])
            n310 = local read "Red Truck Pose"() -> (w499:dbl[])
            n311 = local read "CurrentState"() -> (w480:i32[])
            n312 = local read "CurrentState"() -> (w481:i32[])
            n313 = local read "CurrentState"() -> (w479:i32[])
            n314 = local read "CurrentState"() -> (w470:i32[])
            n315 = local read "CurrentState"() -> (w451:i32[])
            n316 = local read "ID DarkGrey"() -> (w455:u8)
            n317 = local read "CurrentWP"() -> (w486:i32[])
            n318 = local read "CurrentWP"() -> (w492:i32[])
            n319 = local read "CurrentWP"() -> (w491:i32[])
            n320 = local read "CurrentWP"() -> (w468:i32[])
            n321 = local read "CurrentWP"() -> (w453:i32[])
            n322 = local read "ID Black"() -> (w505:u8)
            n323 = local read "ID Blue"() -> (w490:u8)
            n324 = local read "ID Grey"() -> (w466:u8)
            n325 = local read "ID Red"() -> (w494:u8)
            n326 = local read "Vref"() -> (w484:dbl[])
            n327 = local read "Vref"() -> (w483:dbl[])
            n328 = local read "Vref"() -> (w485:dbl[])
            n329 = local read "Vref"() -> (w469:dbl[])
            n330 = local read "Vref"() -> (w452:dbl[])
            n331 = Tick Count (ms)() -> (millisecond timer value=w488:u32)
            n332 = Tick Count (ms)() -> (millisecond timer value=w504:u32)
            n333 = Tick Count (ms)() -> (millisecond timer value=w495:u32)
            n334 = Tick Count (ms)() -> (millisecond timer value=w461:u32)
            n335 = Tick Count (ms)() -> (millisecond timer value=w457:u32)
            n336 = local read "COM  DarkGrey"() -> (w444:T2)
            n337 = local read "COM  Black"() -> (w436:T2)
            n338 = local read "COM  Grey"() -> (w464:T2)
            n339 = local read "COM Blue"() -> (w506:T2)
            n340 = local read "COM  Red"() -> (w440:T2)
            n341 = feedback #1(T6 {"pose"=[0.0, 0.0, 0.0], "totalerror_v"=0.0, "erroSteering"=0.0, "ActualTime"=0.0, "ActualTime 2"=0.0} ("Red feedback init")) -> (w430:T6)
            n342 = call "Controller.vi"("ControllerGains"="ControllerGains Blue", "Current State"=w480, "MyID"=w490, "Pose"=w489, "Feedback elements In"=w430, "CurrentWP"=w486, "Vref"=w484, "Trajectory"=w487, "ActualTime"=w488) -> ("Feedback elements Out"=w431:T12, "v_real"=→"Real Speed Blue":dbl, "Controls"=w507:u8[])  [unwired: 8 in]
            n343 = feedback-in #1(w431) -> ()
            n344 = feedback #2(T6 {"pose"=[0.0, 0.0, 0.0], "totalerror_v"=0.0, "erroSteering"=0.0, "ActualTime"=0.0, "ActualTime 2"=0.0} ("Red feedback init")) -> (w433:T6)
            n345 = call "Controller.vi"("ControllerGains"="ControllerGains Black", "Current State"=w481, "MyID"=w505, "Pose"=w503, "Feedback elements In"=w433, "CurrentWP"=w492, "Vref"=w483, "Trajectory"=w478, "ActualTime"=w504) -> ("Feedback elements Out"=w434:T12, "v_real"=→"Real Speed Black":dbl, "Controls"=w500:u8[])  [unwired: 8 in]
            n346 = feedback-in #2(w434) -> ()
            n347 = feedback #3(T6 {"pose"=[0.0, 0.0, 0.0], "totalerror_v"=0.0, "erroSteering"=0.0, "ActualTime"=0.0, "ActualTime 2"=0.0} ("Red feedback init")) -> (w437:T6)
            n348 = call "Controller.vi"("ControllerGains"="ControllerGains Red", "Current State"=w479, "MyID"=w494, "Pose"=w499, "Feedback elements In"=w437, "CurrentWP"=w491, "Vref"=w485, "Trajectory"=w493, "ActualTime"=w495) -> ("Feedback elements Out"=w438:T12, "v_real"=→"Real Speed Red":dbl, "Controls"=w498:u8[])  [unwired: 8 in]
            n349 = feedback-in #3(w438) -> ()
            n350 = feedback #4(T6 {"pose"=[0.0, 0.0, 0.0], "totalerror_v"=0.0, "erroSteering"=0.0, "ActualTime"=0.0, "ActualTime 2"=0.0} ("Red feedback init")) -> (w472:T6)
            n351 = call "Controller.vi"("ControllerGains"="ControllerGains Grey", "Current State"=w470, "MyID"=w466, "Pose"=w459, "Feedback elements In"=w472, "CurrentWP"=w468, "Vref"=w469, "Trajectory"=w467, "ActualTime"=w461) -> ("Feedback elements Out"=w471:T12, "v_real"=→"Real Speed Grey":dbl, "Controls"=w463:u8[])  [unwired: 8 in]
            n352 = feedback-in #4(w471) -> ()
            n353 = feedback #5(T6 {"pose"=[0.0, 0.0, 0.0], "totalerror_v"=0.0, "erroSteering"=0.0, "ActualTime"=0.0, "ActualTime 2"=0.0} ("Red feedback init")) -> (w441:T6)
            n354 = call "Controller.vi"("ControllerGains"="ControllerGains DarkGrey", "Current State"=w451, "MyID"=w455, "Pose"=w458, "Feedback elements In"=w441, "CurrentWP"=w453, "Vref"=w452, "Trajectory"=w454, "ActualTime"=w457) -> ("Feedback elements Out"=w442:T12, "v_real"=→"Real Speed DarkGrey":dbl, "Controls"=w456:u8[])  [unwired: 8 in]
            n355 = feedback-in #5(w442) -> ()
            n356 = call "CreateSendMSG.vi"("COM Data"=w506, "Controls"=w507) -> ()  [unwired: 18 in]
            n357 = call "CreateSendMSG.vi"("COM Data"=w436, "Controls"=w500) -> ()  [unwired: 18 in]
            n358 = call "CreateSendMSG.vi"("COM Data"=w440, "Controls"=w498) -> ()  [unwired: 18 in]
            n359 = call "CreateSendMSG.vi"("COM Data"=w464, "Controls"=w463) -> ()  [unwired: 18 in]
            n360 = call "CreateSendMSG.vi"("COM Data"=w444, "Controls"=w456) -> ()  [unwired: 18 in]
            n361 = Index Array(array=w507) -> (element #1=→"Blue Steering":u8, element #2=→"Blue Speed":u8)  [unwired: 2 in]
            n362 = Index Array(array=w500) -> (element #1=→"Black Steering":u8, element #2=→"Black Speed":u8)  [unwired: 2 in]
            n363 = Index Array(array=w498) -> (element #1=→"Red Steering":u8, element #2=→"Red Speed":u8)  [unwired: 2 in]
            n364 = Index Array(array=w463) -> (element #1=→"Grey Steering":u8, element #2=→"Grey Speed":u8)  [unwired: 2 in]
            n365 = Index Array(array=w456) -> (element #1=→"DarkGrey Steering":u8, element #2=→"DarkGrey Speed":u8)  [unwired: 2 in]
          }
          frame #6 {
            n366 = local read "Iter"() -> (w515:i32)
            n367 = Quotient & Remainder(x=w515, y=1) -> (x-y*floor(x/y)=w514:i32)  [unwired: 1 out]
            n368 = Equal To 0?(x=w514) -> (x = 0?=w513:bool)
            n369 = local read "Quadcopter"() -> (w510:bool)
            n370 = local read "Visualizer"() -> (w512:bool)
            n371 = And(x=w513, y=w512) -> (x .and. y?=w511:bool)
            n372 = case shown="True" w511 {
              frame False {
              }
              frame True {
                n373 = flat-sequence {
                  frame #0 {
                    n374 = local read "NTrucks"() -> (w554:i32)
                    n375 = Multiply(x=w554, y=3) -> (x*y=w555:i32)
                    n376 = local read "TL Outer Select"() -> (w551:bool)
                    n377 = local read "TL Inner Select"() -> (w552:bool)
                    n378 = local read "Trucks Poses"() -> (w546:dbl[][])
                    n379 = local read "Trailers"() -> (w524:bool[])
                    n380 = global read "Global.vi" "stop"() -> (w545:bool)
                    n381 = Boolean To (0,1)(Boolean=w545) -> (0, 1=w547:i16)
                    n382 = Boolean To (0,1)(Boolean=w551) -> (0, 1=w548:i16)
                    n383 = Boolean To (0,1)(Boolean=w552) -> (0, 1=w549:i16)
                    n384 = Boolean To (0,1)(Boolean=w524) -> (0, 1=w525:i16[])
                    n385 = Reshape Array(w546, w555) -> (w539:dbl[])
                    n386 = local read "Traffic Light Position Outer Lane"() -> (w531:i32)
                    n387 = local read "Traffic Light Position Inner Lane"() -> (w532:i32)
                    n388 = local read "Platooning Distance Scenario"() -> (w530:dbl)
                    n389 = local read "Distance to Master"() -> (w538:dbl[])
                    n390 = local read "StopArrayOuter"() -> (w527:i32[])
                    n391 = local read "StopArrayInner"() -> (w526:i32[])
                    n392 = local read "PlatoonArray"() -> (w528:i32[])
                    n393 = local read "CurrentState"() -> (w535:i32[])
                    n394 = local read "CurrentWP"() -> (w536:i32[])
                    n395 = global read "Global.vi" "RealSpeed"() -> (w534:dbl[])
                    n396 = local read "D2TLFinal"() -> (w537:dbl[])
                    n397 = global read "Global.vi" "MasterID"() -> (w533:i32)
                    n398 = local read "Vref"() -> (w529:dbl[])
                    n399 = Build Array (concatenate)(w547, w548, w549, w531, w532, w533, w530, w534, w535, w536, w537, w538, w529, w528, w527, w526, w525, w539) -> (w550:dbl[])
                    n400 = To Double Precision Float(number=w550) -> (double precision float=w544:dbl[])
                    n401 = Type Cast(x=w544) -> (*(type *) &x=w540:string)  [unwired: 1 in]
                    n402 = local read "Error TCP"() -> (w542:errorcluster)
                    n403 = local read "TCP ID"() -> (w541:refnum<k5>)
                    n404 = TCP Write(connection ID=w541, data in=w540, error in (no error)=w542) -> (error out=w543:errorcluster)  [unwired: 1 in, 2 out]
                    n405 = local write "Error TCP"(w543) -> ()
                  }
                  frame #1 {
                    n406 = local read "ScenarioString"() -> (w558:string)
                    n407 = String Length(string=w558) -> (length=w557:i32)
                    "length" <- w557
                    n408 = To Double Precision Float(number=w557) -> (double precision float=w556:dbl)
                    n409 = Type Cast(x=w556) -> (*(type *) &x=w561:string)  [unwired: 1 in]
                    n410 = local read "Error TCP"() -> (w564:errorcluster)
                    n411 = local read "TCP ID"() -> (w565:refnum<k5>)
                    n412 = TCP Write(connection ID=w565, data in=w561, error in (no error)=w564) -> (connection ID out=w560:refnum<k5>, bytes written=→"bytes written 2":i32, error out=w559:errorcluster)  [unwired: 1 in]
                    n413 = TCP Write(connection ID=w560, data in=w558, error in (no error)=w559) -> (bytes written=→"bytes written 3":i32, error out=w563:errorcluster)  [unwired: 1 in, 1 out]
                    n414 = local write "Error TCP"(w563) -> ()
                  }
                }
              }
            }
            n415 = case shown="True" w510 {
              frame False {
              }
              frame True {
                n416 = global read "Global.vi" "MasterID"() -> (w520:i32)
                n417 = local read "Error TCP_quad"() -> (w522:errorcluster)
                n418 = local read "TCP_quad ID"() -> (w523:refnum<k5>)
                n419 = To Double Precision Float(number=w520) -> (double precision float=w521:dbl)
                n420 = Type Cast(x=w521) -> (*(type *) &x=w519:string)  [unwired: 1 in]
                n421 = TCP Write(connection ID=w523, data in=w519, error in (no error)=w522) -> (connection ID out=w518:refnum<k5>, error out=w517:errorcluster)  [unwired: 1 in, 1 out]
                n422 = local write "TCP_quad ID"(w518) -> ()
                n423 = local write "Error TCP_quad"(w517) -> ()
              }
            }
          }
        }
        n424 = global write "Global.vi" "stop"("stop") -> ()
        n425 = Wait Until Next ms Multiple(millisecond multiple=u32 100) -> ()  [unwired: 1 out]
        "Iter" <- w151
      }
    }
    frame #3 {
      n426 = local read "Visualizer"() -> (w587:bool)
      n427 = local read "Quadcopter"() -> (w584:bool)
      n428 = case shown="True" w584 {
        frame False {
        }
        frame True {
          n429 = local read "Error TCP_quad"() -> (w591:errorcluster)
          n430 = local read "TCP_quad ID"() -> (w592:refnum<k5>)
          n431 = TCP Close Connection(connection ID=w592, error in (no error)=w591) -> ()  [unwired: 1 in, 2 out]
        }
      }
      n432 = case shown="True" w587 {
        frame False {
        }
        frame True {
          n433 = local read "Error TCP"() -> (w602:errorcluster)
          n434 = local read "TCP ID"() -> (w603:refnum<k5>)
          n435 = TCP Close Connection(connection ID=w603, error in (no error)=w602) -> ()  [unwired: 1 in, 2 out]
        }
      }
      n436 = for {
        N: 5 -> [_]
        n437 = local read "COM Blue"() -> (w607:T2)
        n438 = Build Array(u8 127 ("Steering"), u8 127 ("Speed")) -> (w604:u8[])
        n439 = call "CreateSendMSG.vi"("COM Data"=w607, "Controls"=w604) -> ()  [unwired: 18 in]
        n440 = Wait Until Next ms Multiple(millisecond multiple=u32 100) -> ()  [unwired: 1 out]
      }
      n441 = for {
        N: 5 -> [_]
        n442 = local read "COM  Red"() -> (w612:T2)
        n443 = Build Array(u8 127 ("Steering"), u8 127 ("Speed")) -> (w609:u8[])
        n444 = call "CreateSendMSG.vi"("COM Data"=w612, "Controls"=w609) -> ()  [unwired: 18 in]
        n445 = Wait Until Next ms Multiple(millisecond multiple=u32 100) -> ()  [unwired: 1 out]
      }
      n446 = for {
        N: 5 -> [_]
        n447 = local read "COM  Black"() -> (w617:T2)
        n448 = Build Array(u8 127 ("Steering"), u8 127 ("Speed")) -> (w614:u8[])
        n449 = call "CreateSendMSG.vi"("COM Data"=w617, "Controls"=w614) -> ()  [unwired: 18 in]
        n450 = Wait Until Next ms Multiple(millisecond multiple=u32 100) -> ()  [unwired: 1 out]
      }
      n451 = for {
        N: 5 -> [_]
        n452 = local read "COM  Grey"() -> (w600:T2)
        n453 = Build Array(u8 127 ("Steering"), u8 127 ("Speed")) -> (w597:u8[])
        n454 = call "CreateSendMSG.vi"("COM Data"=w600, "Controls"=w597) -> ()  [unwired: 18 in]
        n455 = Wait Until Next ms Multiple(millisecond multiple=u32 100) -> ()  [unwired: 1 out]
      }
      n456 = for {
        N: 5 -> [_]
        (unwired) u32 100 ("millisecond multiple")
        n457 = local read "COM  DarkGrey"() -> (w596:T2)
        n458 = Build Array(u8 127 ("Steering"), u8 127 ("Speed")) -> (w593:u8[])
        n459 = call "CreateSendMSG.vi"("COM Data"=w596, "Controls"=w593) -> ()  [unwired: 18 in]
      }
    }
  }
